vi "Save_PM_BPM_data.vi"(11 "date_time":string) -> ()   [LabVIEW 2017]
uses:
  <userlib>/caLab/Private/Get_PV-1D.vi
  <vilib>/Utility/file.llb/Write To Spreadsheet File (string).vi
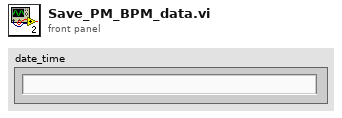
[diagram p1: front panel]
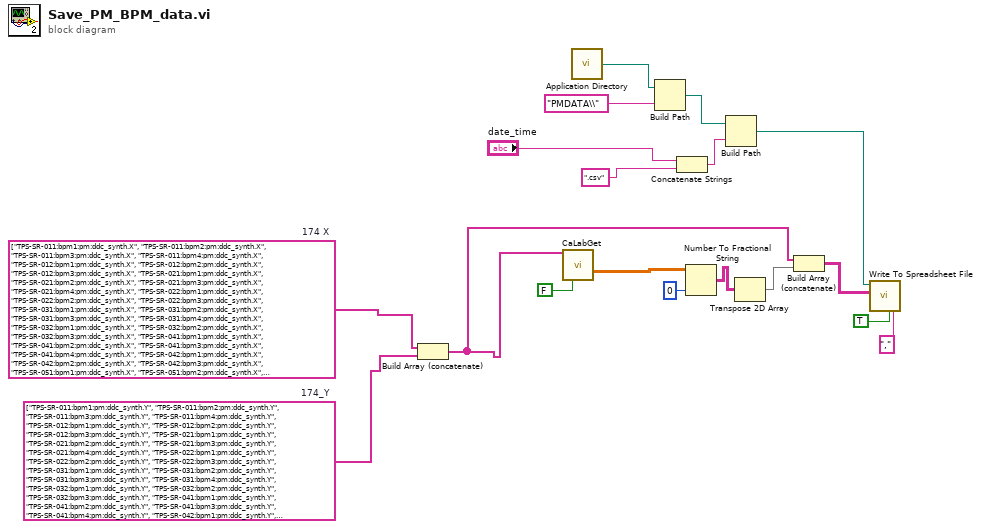
[diagram p0: block diagram]
diagram:
  w14 = string[] ["TPS-SR-011:bpm1:pm:ddc_synth.X", "TPS-SR-011:bpm2:pm:ddc_synth.X", "TPS-SR-011:bpm3:pm:ddc_synth.X", "TPS-SR-011:bpm4:pm:ddc_synth.X", "TPS-SR-012:bpm1:pm:ddc_synth.X", "TPS-SR-012:bpm2:pm:ddc_synth.X", "TPS-SR-012:bpm3:pm:ddc_synth.X", "TPS-SR-021:bpm1:pm:ddc_synth.X", "TPS-SR-021:bpm2:pm:ddc_synth.X", "TPS-SR-021:bpm3:pm:ddc_synth.X", "TPS-SR-021:bpm4:pm:ddc_synth.X", "TPS-SR-022:bpm1:pm:ddc_synth.X", "TPS-SR-022:bpm2:pm:ddc_synth.X", "TPS-SR-022:bpm3:pm:ddc_synth.X", "TPS-SR-031:bpm1:pm:ddc_synth.X", "TPS-SR-031:bpm2:pm:ddc_synth.X", "TPS-SR-031:bpm3:pm:ddc_synth.X", "TPS-SR-031:bpm4:pm:ddc_synth.X", "TPS-SR-032:bpm1:pm:ddc_synth.X", "TPS-SR-032:bpm2:pm:ddc_synth.X", "TPS-SR-032:bpm3:pm:ddc_synth.X", "TPS-SR-041:bpm1:pm:ddc_synth.X", "TPS-SR-041:bpm2:pm:ddc_synth.X", "TPS-SR-041:bpm3:pm:ddc_synth.X", "TPS-SR-041:bpm4:pm:ddc_synth.X", "TPS-SR-042:bpm1:pm:ddc_synth.X", "TPS-SR-042:bpm2:pm:ddc_synth.X", "TPS-SR-042:bpm3:pm:ddc_synth.X", "TPS-SR-051:bpm1:pm:ddc_synth.X", "TPS-SR-051:bpm2:pm:ddc_synth.X", "TPS-SR-051:bpm3:pm:ddc_synth.X", "TPS-SR-051:bpm4:pm:ddc_synth.X", "TPS-SR-052:bpm1:pm:ddc_synth.X", "TPS-SR-052:bpm2:pm:ddc_synth.X", "TPS-SR-052:bpm3:pm:ddc_synth.X", "TPS-SR-061:bpm1:pm:ddc_synth.X", "TPS-SR-061:bpm2:pm:ddc_synth.X", "TPS-SR-061:bpm3:pm:ddc_synth.X", "TPS-SR-061:bpm4:pm:ddc_synth.X", "TPS-SR-062:bpm1:pm:ddc_synth.X", "TPS-SR-062:bpm2:pm:ddc_synth.X", "TPS-SR-062:bpm3:pm:ddc_synth.X", "TPS-SR-071:bpm1:pm:ddc_synth.X", "TPS-SR-071:bpm2:pm:ddc_synth.X", "TPS-SR-071:bpm3:pm:ddc_synth.X", "TPS-SR-071:bpm4:pm:ddc_synth.X", "TPS-SR-072:bpm1:pm:ddc_synth.X", "TPS-SR-072:bpm2:pm:ddc_synth.X", "TPS-SR-072:bpm3:pm:ddc_synth.X", "TPS-SR-081:bpm1:pm:ddc_synth.X", "TPS-SR-081:bpm2:pm:ddc_synth.X", "TPS-SR-081:bpm3:pm:ddc_synth.X", "TPS-SR-081:bpm4:pm:ddc_synth.X", "TPS-SR-082:bpm1:pm:ddc_synth.X", "TPS-SR-082:bpm2:pm:ddc_synth.X", "TPS-SR-082:bpm3:pm:ddc_synth.X", "TPS-SR-091:bpm1:pm:ddc_synth.X", "TPS-SR-091:bpm2:pm:ddc_synth.X", "TPS-SR-091:bpm3:pm:ddc_synth.X", "TPS-SR-091:bpm4:pm:ddc_synth.X", "TPS-SR-092:bpm1:pm:ddc_synth.X", "TPS-SR-092:bpm2:pm:ddc_synth.X", "TPS-SR-092:bpm3:pm:ddc_synth.X", "TPS-SR-101:bpm1:pm:ddc_synth.X", "TPS-SR-101:bpm2:pm:ddc_synth.X", "TPS-SR-101:bpm3:pm:ddc_synth.X", "TPS-SR-101:bpm4:pm:ddc_synth.X", "TPS-SR-102:bpm1:pm:ddc_synth.X", "TPS-SR-102:bpm2:pm:ddc_synth.X", "TPS-SR-102:bpm3:pm:ddc_synth.X", "TPS-SR-111:bpm1:pm:ddc_synth.X", "TPS-SR-111:bpm2:pm:ddc_synth.X", "TPS-SR-111:bpm3:pm:ddc_synth.X", "TPS-SR-111:bpm4:pm:ddc_synth.X", "TPS-SR-112:bpm1:pm:ddc_synth.X", "TPS-SR-112:bpm2:pm:ddc_synth.X", "TPS-SR-112:bpm3:pm:ddc_synth.X", "TPS-SR-121:bpm1:pm:ddc_synth.X", "TPS-SR-121:bpm2:pm:ddc_synth.X", "TPS-SR-121:bpm3:pm:ddc_synth.X", "TPS-SR-121:bpm4:pm:ddc_synth.X", "TPS-SR-122:bpm1:pm:ddc_synth.X", "TPS-SR-122:bpm2:pm:ddc_synth.X", "TPS-SR-122:bpm3:pm:ddc_synth.X", "TPS-SR-131:bpm1:pm:ddc_synth.X", "TPS-SR-131:bpm2:pm:ddc_synth.X", "TPS-SR-131:bpm3:pm:ddc_synth.X", "TPS-SR-131:bpm4:pm:ddc_synth.X", "TPS-SR-132:bpm1:pm:ddc_synth.X", "TPS-SR-132:bpm2:pm:ddc_synth.X", "TPS-SR-132:bpm3:pm:ddc_synth.X", "TPS-SR-141:bpm1:pm:ddc_synth.X", "TPS-SR-141:bpm2:pm:ddc_synth.X", "TPS-SR-141:bpm3:pm:ddc_synth.X", "TPS-SR-141:bpm4:pm:ddc_synth.X", "TPS-SR-142:bpm1:pm:ddc_synth.X", "TPS-SR-142:bpm2:pm:ddc_synth.X", "TPS-SR-142:bpm3:pm:ddc_synth.X", "TPS-SR-151:bpm1:pm:ddc_synth.X", "TPS-SR-151:bpm2:pm:ddc_synth.X", "TPS-SR-151:bpm3:pm:ddc_synth.X", "TPS-SR-151:bpm4:pm:ddc_synth.X", "TPS-SR-152:bpm1:pm:ddc_synth.X", "TPS-SR-152:bpm2:pm:ddc_synth.X", "TPS-SR-152:bpm3:pm:ddc_synth.X", "TPS-SR-161:bpm1:pm:ddc_synth.X", "TPS-SR-161:bpm2:pm:ddc_synth.X", "TPS-SR-161:bpm3:pm:ddc_synth.X", "TPS-SR-161:bpm4:pm:ddc_synth.X", "TPS-SR-162:bpm1:pm:ddc_synth.X", "TPS-SR-162:bpm2:pm:ddc_synth.X", "TPS-SR-162:bpm3:pm:ddc_synth.X", "TPS-SR-171:bpm1:pm:ddc_synth.X", "TPS-SR-171:bpm2:pm:ddc_synth.X", "TPS-SR-171:bpm3:pm:ddc_synth.X", "TPS-SR-171:bpm4:pm:ddc_synth.X", "TPS-SR-172:bpm1:pm:ddc_synth.X", "TPS-SR-172:bpm2:pm:ddc_synth.X", "TPS-SR-172:bpm3:pm:ddc_synth.X", "TPS-SR-181:bpm1:pm:ddc_synth.X", "TPS-SR-181:bpm2:pm:ddc_synth.X", "TPS-SR-181:bpm3:pm:ddc_synth.X", "TPS-SR-181:bpm4:pm:ddc_synth.X", "TPS-SR-182:bpm1:pm:ddc_synth.X", "TPS-SR-182:bpm2:pm:ddc_synth.X", "TPS-SR-182:bpm3:pm:ddc_synth.X", "TPS-SR-191:bpm1:pm:ddc_synth.X", "TPS-SR-191:bpm2:pm:ddc_synth.X", "TPS-SR-191:bpm3:pm:ddc_synth.X", "TPS-SR-191:bpm4:pm:ddc_synth.X", "TPS-SR-192:bpm1:pm:ddc_synth.X", "TPS-SR-192:bpm2:pm:ddc_synth.X", "TPS-SR-192:bpm3:pm:ddc_synth.X", "TPS-SR-201:bpm1:pm:ddc_synth.X", "TPS-SR-201:bpm2:pm:ddc_synth.X", "TPS-SR-201:bpm3:pm:ddc_synth.X", "TPS-SR-201:bpm4:pm:ddc_synth.X", "TPS-SR-202:bpm1:pm:ddc_synth.X", "TPS-SR-202:bpm2:pm:ddc_synth.X", "TPS-SR-202:bpm3:pm:ddc_synth.X", "TPS-SR-211:bpm1:pm:ddc_synth.X", "TPS-SR-211:bpm2:pm:ddc_synth.X", "TPS-SR-211:bpm3:pm:ddc_synth.X", "TPS-SR-211:bpm4:pm:ddc_synth.X", "TPS-SR-212:bpm1:pm:ddc_synth.X", "TPS-SR-212:bpm2:pm:ddc_synth.X", "TPS-SR-212:bpm3:pm:ddc_synth.X", "TPS-SR-221:bpm1:pm:ddc_synth.X", "TPS-SR-221:bpm2:pm:ddc_synth.X", "TPS-SR-221:bpm3:pm:ddc_synth.X", "TPS-SR-221:bpm4:pm:ddc_synth.X", "TPS-SR-222:bpm1:pm:ddc_synth.X", "TPS-SR-222:bpm2:pm:ddc_synth.X", "TPS-SR-222:bpm3:pm:ddc_synth.X", "TPS-SR-231:bpm1:pm:ddc_synth.X", "TPS-SR-231:bpm2:pm:ddc_synth.X", "TPS-SR-231:bpm3:pm:ddc_synth.X", "TPS-SR-231:bpm4:pm:ddc_synth.X", "TPS-SR-232:bpm1:pm:ddc_synth.X", "TPS-SR-232:bpm2:pm:ddc_synth.X", "TPS-SR-232:bpm3:pm:ddc_synth.X", "TPS-SR-241:bpm1:pm:ddc_synth.X", "TPS-SR-241:bpm2:pm:ddc_synth.X", "TPS-SR-241:bpm3:pm:ddc_synth.X", "TPS-SR-241:bpm4:pm:ddc_synth.X", "TPS-SR-242:bpm1:pm:ddc_synth.X", "TPS-SR-242:bpm2:pm:ddc_synth.X", "TPS-SR-242:bpm3:pm:ddc_synth.X"]  # 174 X
  w13 = string[] ["TPS-SR-011:bpm1:pm:ddc_synth.Y", "TPS-SR-011:bpm2:pm:ddc_synth.Y", "TPS-SR-011:bpm3:pm:ddc_synth.Y", "TPS-SR-011:bpm4:pm:ddc_synth.Y", "TPS-SR-012:bpm1:pm:ddc_synth.Y", "TPS-SR-012:bpm2:pm:ddc_synth.Y", "TPS-SR-012:bpm3:pm:ddc_synth.Y", "TPS-SR-021:bpm1:pm:ddc_synth.Y", "TPS-SR-021:bpm2:pm:ddc_synth.Y", "TPS-SR-021:bpm3:pm:ddc_synth.Y", "TPS-SR-021:bpm4:pm:ddc_synth.Y", "TPS-SR-022:bpm1:pm:ddc_synth.Y", "TPS-SR-022:bpm2:pm:ddc_synth.Y", "TPS-SR-022:bpm3:pm:ddc_synth.Y", "TPS-SR-031:bpm1:pm:ddc_synth.Y", "TPS-SR-031:bpm2:pm:ddc_synth.Y", "TPS-SR-031:bpm3:pm:ddc_synth.Y", "TPS-SR-031:bpm4:pm:ddc_synth.Y", "TPS-SR-032:bpm1:pm:ddc_synth.Y", "TPS-SR-032:bpm2:pm:ddc_synth.Y", "TPS-SR-032:bpm3:pm:ddc_synth.Y", "TPS-SR-041:bpm1:pm:ddc_synth.Y", "TPS-SR-041:bpm2:pm:ddc_synth.Y", "TPS-SR-041:bpm3:pm:ddc_synth.Y", "TPS-SR-041:bpm4:pm:ddc_synth.Y", "TPS-SR-042:bpm1:pm:ddc_synth.Y", "TPS-SR-042:bpm2:pm:ddc_synth.Y", "TPS-SR-042:bpm3:pm:ddc_synth.Y", "TPS-SR-051:bpm1:pm:ddc_synth.Y", "TPS-SR-051:bpm2:pm:ddc_synth.Y", "TPS-SR-051:bpm3:pm:ddc_synth.Y", "TPS-SR-051:bpm4:pm:ddc_synth.Y", "TPS-SR-052:bpm1:pm:ddc_synth.Y", "TPS-SR-052:bpm2:pm:ddc_synth.Y", "TPS-SR-052:bpm3:pm:ddc_synth.Y", "TPS-SR-061:bpm1:pm:ddc_synth.Y", "TPS-SR-061:bpm2:pm:ddc_synth.Y", "TPS-SR-061:bpm3:pm:ddc_synth.Y", "TPS-SR-061:bpm4:pm:ddc_synth.Y", "TPS-SR-062:bpm1:pm:ddc_synth.Y", "TPS-SR-062:bpm2:pm:ddc_synth.Y", "TPS-SR-062:bpm3:pm:ddc_synth.Y", "TPS-SR-071:bpm1:pm:ddc_synth.Y", "TPS-SR-071:bpm2:pm:ddc_synth.Y", "TPS-SR-071:bpm3:pm:ddc_synth.Y", "TPS-SR-071:bpm4:pm:ddc_synth.Y", "TPS-SR-072:bpm1:pm:ddc_synth.Y", "TPS-SR-072:bpm2:pm:ddc_synth.Y", "TPS-SR-072:bpm3:pm:ddc_synth.Y", "TPS-SR-081:bpm1:pm:ddc_synth.Y", "TPS-SR-081:bpm2:pm:ddc_synth.Y", "TPS-SR-081:bpm3:pm:ddc_synth.Y", "TPS-SR-081:bpm4:pm:ddc_synth.Y", "TPS-SR-082:bpm1:pm:ddc_synth.Y", "TPS-SR-082:bpm2:pm:ddc_synth.Y", "TPS-SR-082:bpm3:pm:ddc_synth.Y", "TPS-SR-091:bpm1:pm:ddc_synth.Y", "TPS-SR-091:bpm2:pm:ddc_synth.Y", "TPS-SR-091:bpm3:pm:ddc_synth.Y", "TPS-SR-091:bpm4:pm:ddc_synth.Y", "TPS-SR-092:bpm1:pm:ddc_synth.Y", "TPS-SR-092:bpm2:pm:ddc_synth.Y", "TPS-SR-092:bpm3:pm:ddc_synth.Y", "TPS-SR-101:bpm1:pm:ddc_synth.Y", "TPS-SR-101:bpm2:pm:ddc_synth.Y", "TPS-SR-101:bpm3:pm:ddc_synth.Y", "TPS-SR-101:bpm4:pm:ddc_synth.Y", "TPS-SR-102:bpm1:pm:ddc_synth.Y", "TPS-SR-102:bpm2:pm:ddc_synth.Y", "TPS-SR-102:bpm3:pm:ddc_synth.Y", "TPS-SR-111:bpm1:pm:ddc_synth.Y", "TPS-SR-111:bpm2:pm:ddc_synth.Y", "TPS-SR-111:bpm3:pm:ddc_synth.Y", "TPS-SR-111:bpm4:pm:ddc_synth.Y", "TPS-SR-112:bpm1:pm:ddc_synth.Y", "TPS-SR-112:bpm2:pm:ddc_synth.Y", "TPS-SR-112:bpm3:pm:ddc_synth.Y", "TPS-SR-121:bpm1:pm:ddc_synth.Y", "TPS-SR-121:bpm2:pm:ddc_synth.Y", "TPS-SR-121:bpm3:pm:ddc_synth.Y", "TPS-SR-121:bpm4:pm:ddc_synth.Y", "TPS-SR-122:bpm1:pm:ddc_synth.Y", "TPS-SR-122:bpm2:pm:ddc_synth.Y", "TPS-SR-122:bpm3:pm:ddc_synth.Y", "TPS-SR-131:bpm1:pm:ddc_synth.Y", "TPS-SR-131:bpm2:pm:ddc_synth.Y", "TPS-SR-131:bpm3:pm:ddc_synth.Y", "TPS-SR-131:bpm4:pm:ddc_synth.Y", "TPS-SR-132:bpm1:pm:ddc_synth.Y", "TPS-SR-132:bpm2:pm:ddc_synth.Y", "TPS-SR-132:bpm3:pm:ddc_synth.Y", "TPS-SR-141:bpm1:pm:ddc_synth.Y", "TPS-SR-141:bpm2:pm:ddc_synth.Y", "TPS-SR-141:bpm3:pm:ddc_synth.Y", "TPS-SR-141:bpm4:pm:ddc_synth.Y", "TPS-SR-142:bpm1:pm:ddc_synth.Y", "TPS-SR-142:bpm2:pm:ddc_synth.Y", "TPS-SR-142:bpm3:pm:ddc_synth.Y", "TPS-SR-151:bpm1:pm:ddc_synth.Y", "TPS-SR-151:bpm2:pm:ddc_synth.Y", "TPS-SR-151:bpm3:pm:ddc_synth.Y", "TPS-SR-151:bpm4:pm:ddc_synth.Y", "TPS-SR-152:bpm1:pm:ddc_synth.Y", "TPS-SR-152:bpm2:pm:ddc_synth.Y", "TPS-SR-152:bpm3:pm:ddc_synth.Y", "TPS-SR-161:bpm1:pm:ddc_synth.Y", "TPS-SR-161:bpm2:pm:ddc_synth.Y", "TPS-SR-161:bpm3:pm:ddc_synth.Y", "TPS-SR-161:bpm4:pm:ddc_synth.Y", "TPS-SR-162:bpm1:pm:ddc_synth.Y", "TPS-SR-162:bpm2:pm:ddc_synth.Y", "TPS-SR-162:bpm3:pm:ddc_synth.Y", "TPS-SR-171:bpm1:pm:ddc_synth.Y", "TPS-SR-171:bpm2:pm:ddc_synth.Y", "TPS-SR-171:bpm3:pm:ddc_synth.Y", "TPS-SR-171:bpm4:pm:ddc_synth.Y", "TPS-SR-172:bpm1:pm:ddc_synth.Y", "TPS-SR-172:bpm2:pm:ddc_synth.Y", "TPS-SR-172:bpm3:pm:ddc_synth.Y", "TPS-SR-181:bpm1:pm:ddc_synth.Y", "TPS-SR-181:bpm2:pm:ddc_synth.Y", "TPS-SR-181:bpm3:pm:ddc_synth.Y", "TPS-SR-181:bpm4:pm:ddc_synth.Y", "TPS-SR-182:bpm1:pm:ddc_synth.Y", "TPS-SR-182:bpm2:pm:ddc_synth.Y", "TPS-SR-182:bpm3:pm:ddc_synth.Y", "TPS-SR-191:bpm1:pm:ddc_synth.Y", "TPS-SR-191:bpm2:pm:ddc_synth.Y", "TPS-SR-191:bpm3:pm:ddc_synth.Y", "TPS-SR-191:bpm4:pm:ddc_synth.Y", "TPS-SR-192:bpm1:pm:ddc_synth.Y", "TPS-SR-192:bpm2:pm:ddc_synth.Y", "TPS-SR-192:bpm3:pm:ddc_synth.Y", "TPS-SR-201:bpm1:pm:ddc_synth.Y", "TPS-SR-201:bpm2:pm:ddc_synth.Y", "TPS-SR-201:bpm3:pm:ddc_synth.Y", "TPS-SR-201:bpm4:pm:ddc_synth.Y", "TPS-SR-202:bpm1:pm:ddc_synth.Y", "TPS-SR-202:bpm2:pm:ddc_synth.Y", "TPS-SR-202:bpm3:pm:ddc_synth.Y", "TPS-SR-211:bpm1:pm:ddc_synth.Y", "TPS-SR-211:bpm2:pm:ddc_synth.Y", "TPS-SR-211:bpm3:pm:ddc_synth.Y", "TPS-SR-211:bpm4:pm:ddc_synth.Y", "TPS-SR-212:bpm1:pm:ddc_synth.Y", "TPS-SR-212:bpm2:pm:ddc_synth.Y", "TPS-SR-212:bpm3:pm:ddc_synth.Y", "TPS-SR-221:bpm1:pm:ddc_synth.Y", "TPS-SR-221:bpm2:pm:ddc_synth.Y", "TPS-SR-221:bpm3:pm:ddc_synth.Y", "TPS-SR-221:bpm4:pm:ddc_synth.Y", "TPS-SR-222:bpm1:pm:ddc_synth.Y", "TPS-SR-222:bpm2:pm:ddc_synth.Y", "TPS-SR-222:bpm3:pm:ddc_synth.Y", "TPS-SR-231:bpm1:pm:ddc_synth.Y", "TPS-SR-231:bpm2:pm:ddc_synth.Y", "TPS-SR-231:bpm3:pm:ddc_synth.Y", "TPS-SR-231:bpm4:pm:ddc_synth.Y", "TPS-SR-232:bpm1:pm:ddc_synth.Y", "TPS-SR-232:bpm2:pm:ddc_synth.Y", "TPS-SR-232:bpm3:pm:ddc_synth.Y", "TPS-SR-241:bpm1:pm:ddc_synth.Y", "TPS-SR-241:bpm2:pm:ddc_synth.Y", "TPS-SR-241:bpm3:pm:ddc_synth.Y", "TPS-SR-241:bpm4:pm:ddc_synth.Y", "TPS-SR-242:bpm1:pm:ddc_synth.Y", "TPS-SR-242:bpm2:pm:ddc_synth.Y", "TPS-SR-242:bpm3:pm:ddc_synth.Y"]  # 174_Y
  n1 = Build Array (concatenate)(w14, w13) -> (w10:string[])
  n2 = call-poly <userlib>:"CaLabGet.vi"("PV Names"=w10, "NoMDEL(F)"=FALSE) -> ("Value Array (number)"=w12:dbl[][])  [unwired: 7 in, 6 out]
  n3 = call <vilib>:"Application Directory.vi"() -> ("Application Directory"=w18:path)
  n4 = Build Path(base path=w18, name or relative path="PMDATA\\") -> (appended path=w5:path)
  n5 = Concatenate Strings("date_time", ".csv" ("name or relative path")) -> (w3:string)
  n6 = Number To Fractional String(number=w12, precision (6)=i16 0) -> (F-format string=w8:string[][])  [unwired: 2 in]
  n7 = Build Path(base path=w5, name or relative path=w3) -> (appended path=w4:path)
  n8 = Transpose 2D Array(2D array=w8) -> (transposed array=w7:string[][])
  n9 = Build Array (concatenate)(w10, w7) -> (w9:string[][])
  n10 = call-poly <vilib>:"Write To Spreadsheet File.vi"("delimiter (\\t)"="," ("delimiter (\\t)"), "transpose? (no:F)"=TRUE, "2D data"=w9, "file path (dialog if empty)"=w4) -> ()  [unwired: 4 in, 1 out]
